vi "qDSP.vi"(0 "System no.":i32=1 min=1 max=4 step=1, 3 "Invert order?":bool, 5 "error in":errorcluster) -> (14 "Displayed axes":string[](array[string]), 19 "error out":errorcluster)   [LabVIEW 2026]
doc: "Replies which axes are displayed on the controller screen.\n\nC-702: Invert order should be TRUE\nC-848: Invert order should be TRUE\nC-880: Invert order should be TRUE"
uses:
  Communication/Global1.vi
panel:
  # "Replies which axes are displayed on the controller screen."
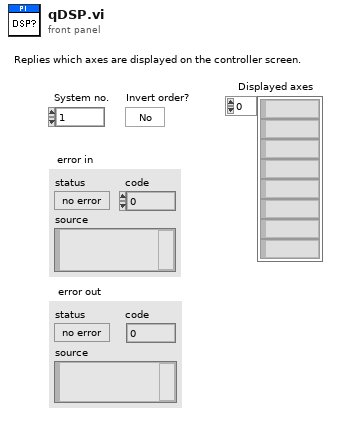
[diagram p1: front panel]
types:
  T1 = typedef "Syntax.ctl" = enum16{"GCS 1.0", "GCS 2.0", "GCS 3.0"}
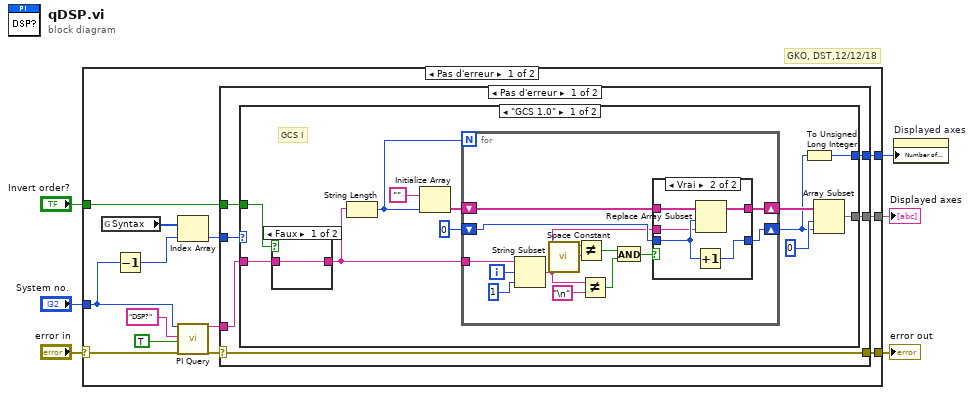
[diagram p0: block diagram]
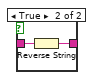
[diagram p2: hidden frame]
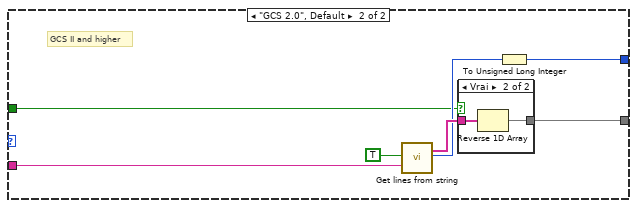
[diagram p4: hidden frame]
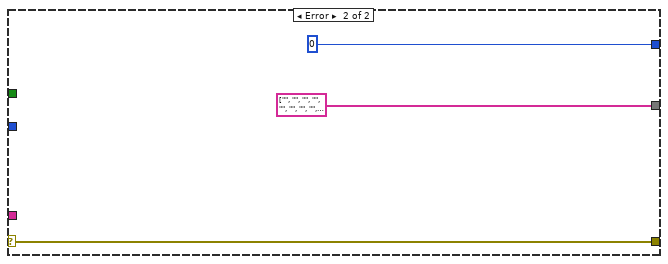
[diagram p6: hidden frame]
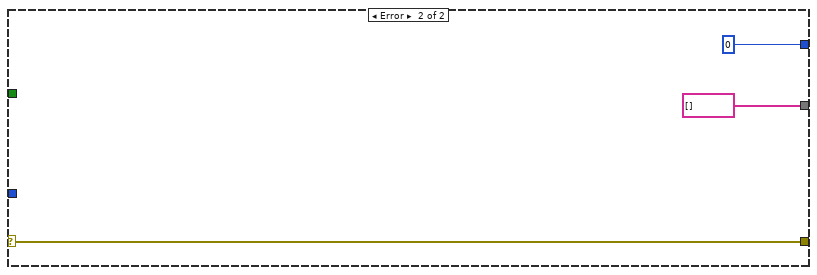
[diagram p7: hidden frame]
diagram:
  # "GKO, DST,12/12/18"
  n1 = case shown="Pas d'erreur" "error in" {
    selector: "error in" -> [w10 w76]
    tunnel: [w17 0 ("Array size out")] -> w6
    tunnel: [w16 string[] [] ("Conn. Axes 2")] -> w5
    tunnel: "System no." -> [w13 _]
    tunnel: [w7 w76] -> w3
    tunnel: "Invert order?" -> [w11 _]
    frame No Error {
      n2 = global read "Global1.vi" "Syntax"() -> (w14:T1[])
      n3 = Decrement(x=w13) -> (x-1=w15:i32)
      n4 = Index Array(array=w14, index=w15) -> (element=w9:T1)
      n5 = call "PI Query.vi"("System no."=w13, "String to send"="DSP?", "Attach termination char.?"=TRUE ("Attach Linefeed?"), "error in"=w10) -> ("String read"=w12:string, "error out"=w8:errorcluster)  [unwired: 3 in, 11 out]
      n6 = case shown="Pas d'erreur" w8 {
        selector: w8 -> [w20 w72]
        tunnel: w12 -> [w22 _]
        tunnel: [w25 u32 0] -> w17
        tunnel: [w24 string[] ["", "", "", "", "", "", "", "", "", "", "", "", "", "", "", "", "", "", "", "", "", "", "", "", "", "", ""] ("Conn. Axes 2")] -> w16
        tunnel: w11 -> [w23 _]
        tunnel: w9 -> [w21 _]
        tunnel: [w20 w72] -> w7
        frame No Error {
          n7 = case shown="\"GCS 1.0\"" w21 {
            tunnel: [w26 w61] -> w25
            tunnel: [w31 w63] -> w24
            tunnel: w23 -> [w29 w62]
            tunnel: w22 -> [w28 w65]
            frame "GCS 1.0" {
              # "GCS I"
              n8 = case shown="Faux" w29 {
                tunnel: w28 -> [w38 w40]
                tunnel: [w38 w39] -> w30
                frame False {
                }
                frame True {
                  n9 = Reverse String(1:w40) -> (0:w39:string)
                }
              }
              n10 = String Length(string=w30) -> (length=w36:i32)
              n11 = Initialize Array("" ("Element Data"), w36) -> (w34:string[])
              n12 = for {
                N: w36 -> [_]
                tunnel: w30 -> [w53]
                shift-right: [w46] -> w32
                shift-left: w34 -> [w47]
                shift-right: [w49] -> w27
                shift-left: 0 -> [w48]
                i -> [w51]
                n13 = String Subset(string=w53, offset (0)=w51, length (rest)=1 ("length")) -> (substring=w45:string)
                n14 = call <vilib>:"Space Constant.vi"() -> ("String"=w50:string)
                n15 = Not Equal?(x=w45, y=w50) -> (x != y?=w43:bool)
                n16 = Not Equal?(x=w45, y="\n") -> (x != y?=w42:bool)
                n17 = And(x=w43, y=w42) -> (x .and. y?=w41:bool)
                n18 = case shown="Vrai" w41 {
                  tunnel: [w55 w60] -> w49
                  tunnel: w48 -> [w55 w58]
                  tunnel: w47 -> [w54 w59]
                  tunnel: w45 -> [_ w57]
                  tunnel: [w54 w56] -> w46
                  frame False {
                  }
                  frame True {
                    n19 = Increment(x=w58) -> (x+1=w60:i32)
                    n20 = Replace Array Subset(array=w59, new element=w57, index=w58) -> (w56:string[])
                  }
                }
              }
              n21 = To Unsigned Long Integer(number=w27) -> (unsigned 32bit integer=w26:u32)
              n22 = Array Subset(array=w32, index=0 ("Array Index"), length=w27) -> (w31:string[])
            }
            frame "GCS 2.0", Default {
              # "GCS II and higher"
              n23 = call "Get lines from string.vi"("Cut spaces?"=TRUE, "Input string"=w65) -> ("Strings"=w66:string[], "Array size out"=w64:i32)  [unwired: 1 in, 15 out]
              n24 = case shown="Vrai" w62 {
                tunnel: w66 -> [w68 w70]
                tunnel: [w68 w69] -> w63
                frame False {
                }
                frame True {
                  n25 = Reverse 1D Array(array=w70) -> (reversed array=w69:string[])
                }
              }
              n26 = To Unsigned Long Integer(number=w64) -> (unsigned 32bit integer=w61:u32)
            }
          }
        }
        frame Error {
        }
      }
    }
    frame Error {
    }
  }
  "error out" <- w3
  "Displayed axes" <- w5
  n27 = property on="Displayed axes" class="Tabl (strict)"("Number of Rows"=w6) -> ()  [unwired: 2 in, 2 out]
